vi "testFlushTelToDds.vi"(8 "error in (no error)":errorcluster) -> (0 "error out":errorcluster)   [LabVIEW 2018]
doc: "Test the flushTel.vi with queueTelToDds option."
uses:
  src/TcpServer/TcpServer.lvclass
  src/TcpServer/TcpServer.lvclass/TcpServer.ctl
  src/TcpServerBase/TcpServerBase.lvclass/TcpServerBase.ctl
  src/TcpServerTel/TcpServerTel.lvclass
  home/pcortes/github/ts_labview_tcp_json/src/TcpServerBase/TcpServerBase.lvclass
  <vilib>/addons/_JKI Toolkits/Caraya/classes/Assert/Assert Equal Value_Variant.vi
  <vilib>/addons/_JKI Toolkits/Caraya/classes/Test/Test.lvclass
  <vilib>/addons/_JKI Toolkits/Caraya/classes/Assert/Assert.lvclass
  src/TcpServerBase/TcpServerBase.lvclass
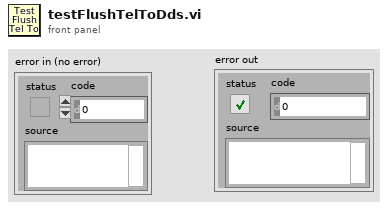
[diagram p1: front panel]
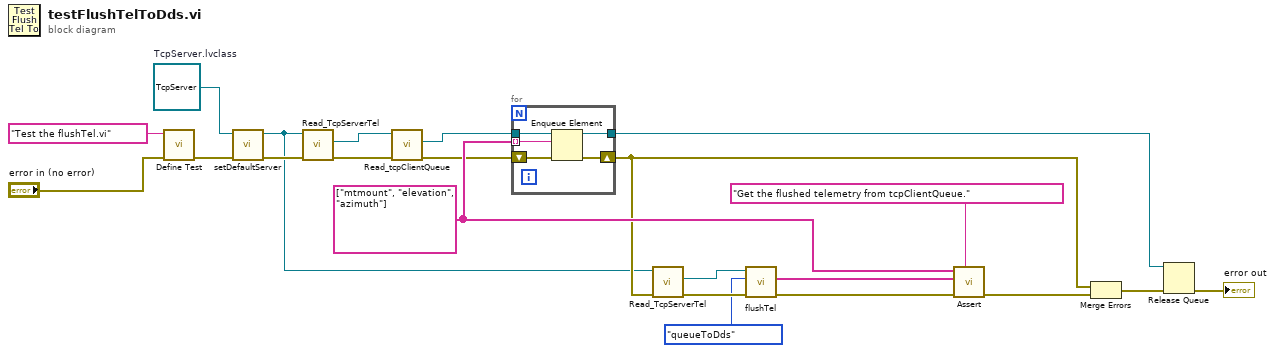
[diagram p0: block diagram]
diagram:
  w11 = string[] ["mtmount", "elevation", "azimuth"]
  w7 = refnum<class "TcpServer.lvclass"> refnum  # TcpServer.lvclass
  n1 = call <vilib>:"Define Test.vi"("error in (no error)"="error in (no error)", "Label (VI Title)"="Test the flushTel.vi") -> ("error out"=w21:errorcluster)  [unwired: 9 in]
  n2 = call "setDefaultServer.vi"("error in (no error)"=w21, "TcpServer.lvclass"=w7) -> ("error out"=w14:errorcluster, "tcpServer out"=w6:refnum<class "TcpServer.lvclass">)  [unwired: 8 in]
  n3 = call "Read_TcpServerTel.vi"("error in (no error)"=w14, "TcpServer in"=w6) -> ("error out"=w3:errorcluster, "TcpServerTel.lvclass"=w4:refnum<class "TcpServerTel.lvclass">)  [unwired: 7 in, 1 out]
  n4 = call "Read_tcpClientQueue.vi"("error in (no error)"=w3, "TcpServerBase in"=w4) -> ("error out"=w2:errorcluster, "tcpClientQueue"=w1:refnum<queue>)  [unwired: 7 in, 1 out]
  n5 = for {
    tunnel: w11 -> [w26] mode=indexing
    tunnel: [w24] -> w15
    shift-right: [w25] -> w10
    shift-left: w2 -> [w27]
    tunnel: w1 -> [w23]
    n6 = Enqueue Element(queue=w23, element=w26, error in (no error)=w27) -> (queue out=w24:refnum<queue>, error out=w25:errorcluster)  [unwired: 1 in, 1 out]
  }
  n7 = call "Read_TcpServerTel.vi"("error in (no error)"=w10, "TcpServer in"=w6) -> ("error out"=w9:errorcluster, "TcpServerTel.lvclass"=w8:refnum<class "TcpServerTel.lvclass">)  [unwired: 7 in, 1 out]
  n8 = call "flushTel.vi"("error in (no error)"=w9, "queueName"=enum16{"queueFromDds", "queueToDds"}."queueToDds", "tcpServerTel in"=w8) -> ("error out"=w13:errorcluster, "telemetry flushed"=w12:string[])  [unwired: 6 in, 1 out]
  n9 = call-poly <vilib>:"Assert.vi"("Label"="Get the flushed telemetry from tcpClientQueue.", "error in (no error)"=w13, "Y"=w12, "X"=w11) -> ("error out"=w18:errorcluster)  [unwired: 7 in]
  n10 = Merge Errors(w10, w18) -> (w16:errorcluster)
  n11 = Release Queue(queue=w15, error in (no error)=w16) -> (error out=→"error out":errorcluster)  [unwired: 1 in, 2 out]
